vi "ValveControl.vi"(0 "error in":errorcluster, 1 "SV5":u16(ring) items=["FIO0", "FIO1", "FIO2", "FIO3", "FIO4", "FIO5", "FIO6", "FIO7", "EIO0", "EIO1", "EIO2", "EIO3", "EIO4", "EIO5", "EIO6", "EIO7", "CIO0", "CIO1", "CIO2", "CIO3", "MIO0", "MIO1", "MIO2"], 2 "SV6":u16(ring) items=["FIO0", "FIO1", "FIO2", "FIO3", "FIO4", "FIO5", "FIO6", "FIO7", "EIO0", "EIO1", "EIO2", "EIO3", "EIO4", "EIO5", "EIO6", "EIO7", "CIO0", "CIO1", "CIO2", "CIO3", "MIO0", "MIO1", "MIO2"], 4 "Solenoid States":bool[](array[boolean]), 5 "SV3":u16(ring) items=["FIO0", "FIO1", "FIO2", "FIO3", "FIO4", "FIO5", "FIO6", "FIO7", "EIO0", "EIO1", "EIO2", "EIO3", "EIO4", "EIO5", "EIO6", "EIO7", "CIO0", "CIO1", "CIO2", "CIO3", "MIO0", "MIO1", "MIO2"], 6 "SV4":u16(ring) items=["FIO0", "FIO1", "FIO2", "FIO3", "FIO4", "FIO5", "FIO6", "FIO7", "EIO0", "EIO1", "EIO2", "EIO3", "EIO4", "EIO5", "EIO6", "EIO7", "CIO0", "CIO1", "CIO2", "CIO3", "MIO0", "MIO1", "MIO2"], 7 "Handle In":i32, 8 "SV0":u16(ring) items=["FIO0", "FIO1", "FIO2", "FIO3", "FIO4", "FIO5", "FIO6", "FIO7", "EIO0", "EIO1", "EIO2", "EIO3", "EIO4", "EIO5", "EIO6", "EIO7", "CIO0", "CIO1", "CIO2", "CIO3", "MIO0", "MIO1", "MIO2"], 9 "SV1":u16(ring) items=["FIO0", "FIO1", "FIO2", "FIO3", "FIO4", "FIO5", "FIO6", "FIO7", "EIO0", "EIO1", "EIO2", "EIO3", "EIO4", "EIO5", "EIO6", "EIO7", "CIO0", "CIO1", "CIO2", "CIO3", "MIO0", "MIO1", "MIO2"], 10 "SV2":u16(ring) items=["FIO0", "FIO1", "FIO2", "FIO3", "FIO4", "FIO5", "FIO6", "FIO7", "EIO0", "EIO1", "EIO2", "EIO3", "EIO4", "EIO5", "EIO6", "EIO7", "CIO0", "CIO1", "CIO2", "CIO3", "MIO0", "MIO1", "MIO2"]) -> (3 "error out":errorcluster[](array[cluster]))   [LabVIEW 2021]
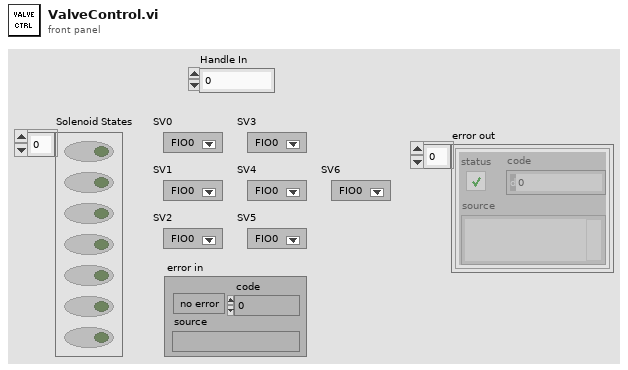
[diagram p1: front panel]
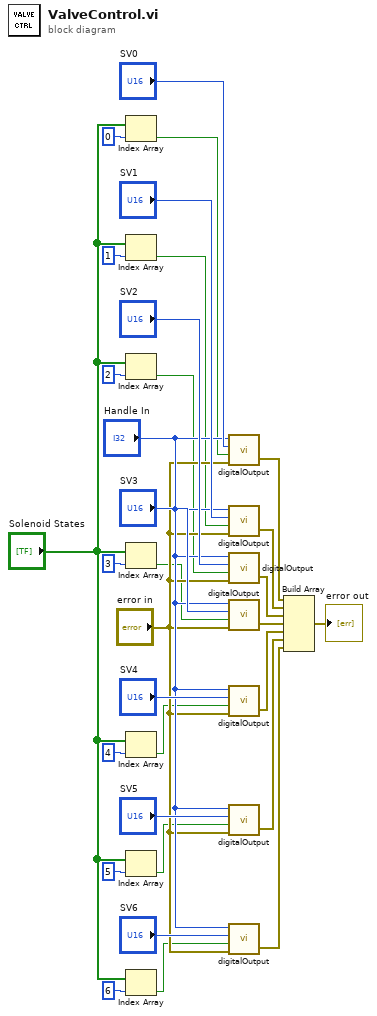
[diagram p0: block diagram]
diagram:
  n1 = Index Array(array="Solenoid States", index=0) -> (element=w7:bool)
  n2 = Index Array(array="Solenoid States", index=1) -> (element=w6:bool)
  n3 = Index Array(array="Solenoid States", index=2) -> (element=w5:bool)
  n4 = Index Array(array="Solenoid States", index=3) -> (element=w4:bool)
  n5 = Index Array(array="Solenoid States", index=4) -> (element=w3:bool)
  n6 = Index Array(array="Solenoid States", index=5) -> (element=w2:bool)
  n7 = Index Array(array="Solenoid States", index=6) -> (element=w1:bool)
  n8 = call "digitalOutput.vi"("error in"="error in", "State"=w7, "Channel"="SV0", "Handle In"="Handle In") -> ("error out"=w23:errorcluster)  [unwired: 1 out]
  n9 = call "digitalOutput.vi"("error in"="error in", "State"=w6, "Channel"="SV1", "Handle In"="Handle In") -> ("error out"=w22:errorcluster)  [unwired: 1 out]
  n10 = call "digitalOutput.vi"("error in"="error in", "State"=w5, "Channel"="SV2", "Handle In"="Handle In") -> ("error out"=w21:errorcluster)  [unwired: 1 out]
  n11 = call "digitalOutput.vi"("error in"="error in", "State"=w4, "Channel"="SV3", "Handle In"="Handle In") -> ("error out"=w20:errorcluster)  [unwired: 1 out]
  n12 = call "digitalOutput.vi"("error in"="error in", "State"=w3, "Channel"="SV4", "Handle In"="Handle In") -> ("error out"=w19:errorcluster)  [unwired: 1 out]
  n13 = call "digitalOutput.vi"("error in"="error in", "State"=w2, "Channel"="SV5", "Handle In"="Handle In") -> ("error out"=w18:errorcluster)  [unwired: 1 out]
  n14 = call "digitalOutput.vi"("error in"="error in", "State"=w1, "Channel"="SV6", "Handle In"="Handle In") -> ("error out"=w17:errorcluster)  [unwired: 1 out]
  n15 = Build Array(w23, w22, w21, w20, w19, w18, w17) -> (→"error out":errorcluster[])
